vi "State_Machine.vi"() -> ()   [LabVIEW 2022 SP3]
uses:
  <vilib>/numeric/Random Number (Range) I64.vi
  <vilib>/numeric/sub_Random U32.vi
panel:
  out "Rand":dbl
  out "Message":string
  in  "OK Button":bool
  in  "Guess":dbl
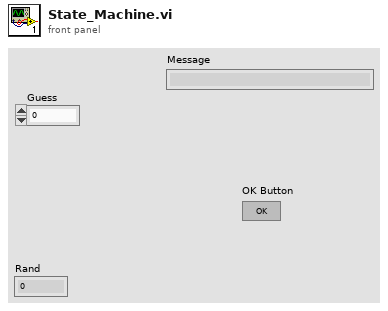
[diagram p1: front panel]
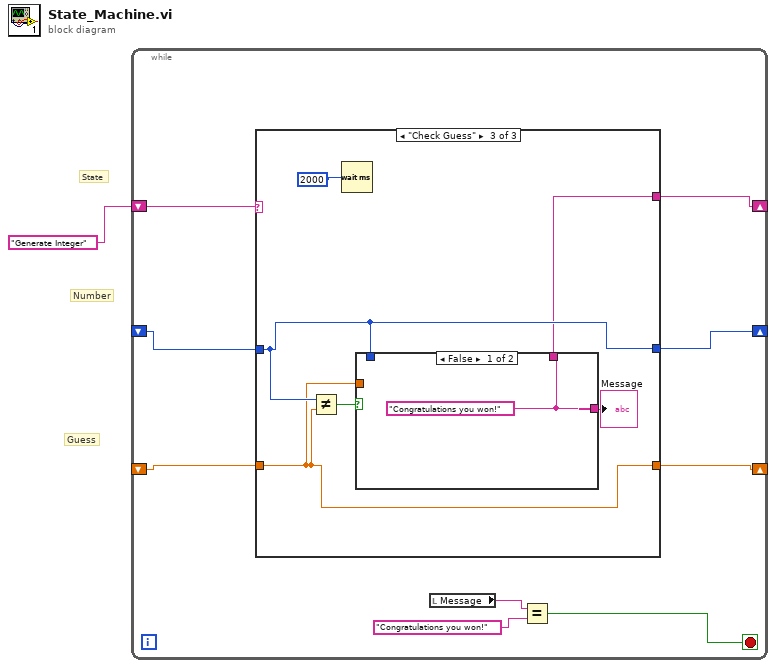
[diagram p0: block diagram]
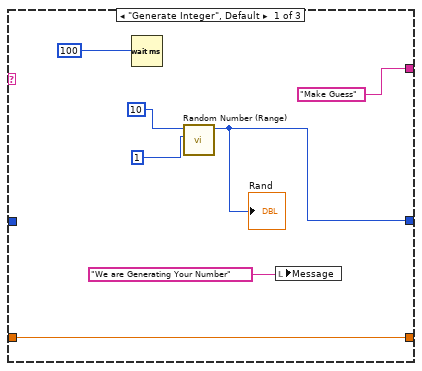
[diagram p2: hidden frame]
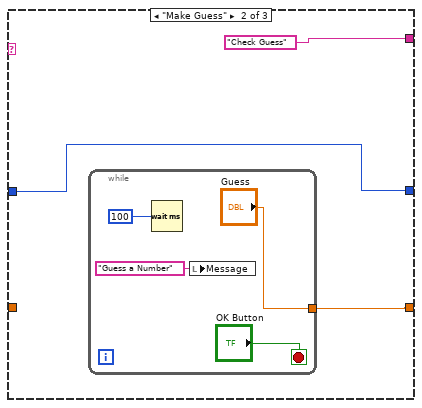
[diagram p3: hidden frame]
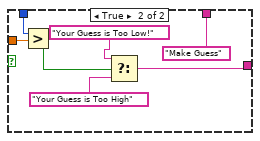
[diagram p4: hidden frame]
diagram:
  # "Guess"
  # "Number"
  # "State"
  n1 = while {
    shift-right: [w7] -> _
    shift-left: "Generate Integer" -> [w10]
    shift-right: [w9] -> _
    shift-left: _ -> [w6]
    shift-right: [w8] -> _
    shift-left: _ -> [w5]
    stop <- w2 stop-if-true
    n2 = case shown="\"Check Guess\"" w10 {
      tunnel: w6 -> [_ w19 w27]
      tunnel: [w11 w19 w27] -> w9
      tunnel: [w15 w20 w26] -> w8
      tunnel: w5 -> [w15 _ w26]
      tunnel: ["Make Guess" "Check Guess" w25] -> w7
      frame "Generate Integer", Default {
        n3 = Wait (ms)(milliseconds to wait=100) -> ()  [unwired: 1 out]
        n4 = call-poly <vilib>:"Random Number (Range).vi"("lower bound (-100)"=1, "upper bound (100)"=10) -> ("number"=w11:i64)  [unwired: 9 in]
        "Rand" <- w11
        n5 = local write "Message"("We are Generating Your Number") -> ()
      }
      frame "Make Guess" {
        n6 = while {
          tunnel: ["Guess"] -> w20
          stop <- "OK Button" stop-if-true
          n7 = Wait (ms)(milliseconds to wait=100) -> ()  [unwired: 1 out]
          n8 = local write "Message"("Guess a Number") -> ()
        }
      }
      frame "Check Guess" {
        n9 = Not Equal?(x=w27, y=w26) -> (x != y?=w29:bool)
        n10 = Wait (ms)(milliseconds to wait=2000) -> ()  [unwired: 1 out]
        n11 = case shown="False" w29 {
          tunnel: [w31 w36] -> w28
          tunnel: w27 -> [_ w38]
          tunnel: w26 -> [_ w37]
          tunnel: [w31 "Make Guess"] -> w25
          frame False {
            w31 = "Congratulations you won!"
          }
          frame True {
            n12 = Greater?(x=w38, y=w37) -> (0:w35:bool)
            n13 = Select(t="Your Guess is Too Low!", s=w35, f="Your Guess is Too High") -> (s? t:f=w36:string)
          }
        }
        "Message" <- w28
      }
    }
    n14 = local read "Message"() -> (w3:string)
    n15 = Equal?(x=w3, y="Congratulations you won!") -> (x = y?=w2:bool)
  }
